vi "Wait-for-action-deposition.vi"(8 "error in (no error)":errorcluster, 11 "Object ref in":T2) -> (0 "error out":errorcluster, 2 "Action":T1=enum."Load deposition", 3 "Object ref out":T2)   [LabVIEW 2013, in "SLMControl.lvlib" / "SC-Main.lvclass"]
uses:
  SC-Main.lvclass
  Object-reference.ctl
  Deposition-actions.ctl
  SC-Main.lvclass/SC-Main.ctl
  Read Deposition queue.vi
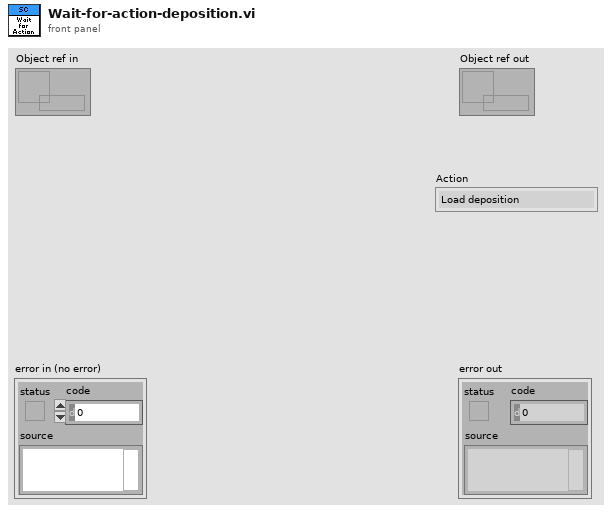
[diagram p1: front panel]
types:
  T1 = typedef "SLMControl.lvlib/SC-Main.lvclass/Deposition-actions.ctl" = enum16{"Idle", "Activate", "Load deposition", "Launch deposition", "Wait for deposition end", "Signal lasing", "Abort", "Reset", "Exit"}
  T2 = typedef "SLMControl.lvlib/SC-Main.lvclass/Object-reference.ctl" = refnum<data-value>
  T3 = typedef "BeamControl.lvlib/BC-Main.lvclass/Deposition-actions.ctl" = enum16{"Idle", "Activate", "Load deposition", "Launch deposition", "Wait for deposition end", "Signal lasing", "Abort", "Reset", "Exit"}
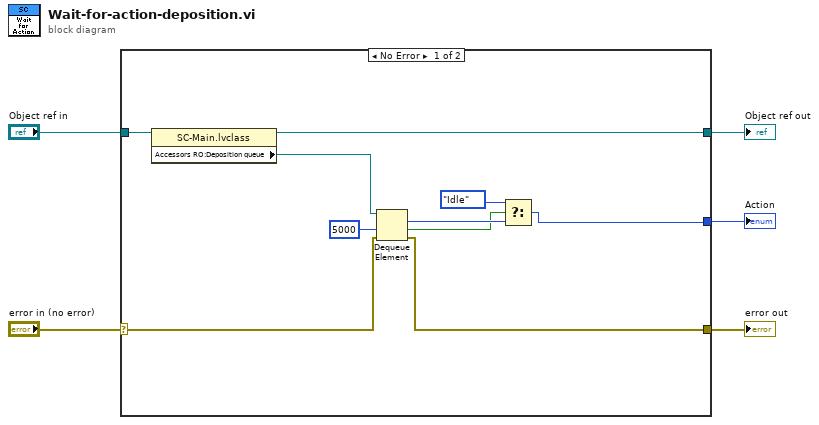
[diagram p0: block diagram]
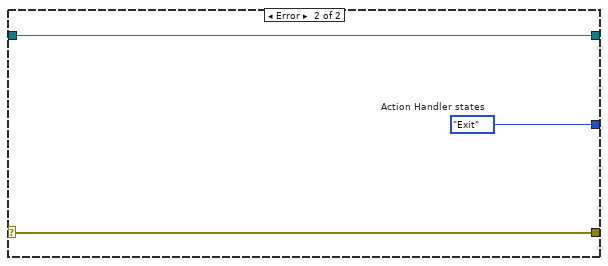
[diagram p2: hidden frame]
diagram:
  n1 = case shown="No Error" "error in (no error)" {
    selector: "error in (no error)" -> [w13 w18]
    tunnel: [w12 w18] -> w4
    tunnel: [w14 w17] -> w2
    tunnel: "Object ref in" -> [w15 w17]
    tunnel: [w6 w16] -> w1
    frame No Error {
      n2 = property class="SC-Main.lvclass"(reference=w15) -> (reference out=w14:T2, "Accessors RO:Deposition queue"=w11:refnum<queue>)  [unwired: 1 in, 1 out]
      n3 = Dequeue Element(queue=w11, timeout in ms (-1)=5000, error in (no error)=w13) -> (element=w9:T3, timed out?=w8:bool, error out=w12:errorcluster)  [unwired: 1 out]
      n4 = Select(t=Deposition-actions."Idle" ("Next execution"), s=w8, f=w9) -> (s? t:f=w6:T3)
    }
    frame Error {
      w16 = Deposition-actions."Exit"  # Action Handler states
    }
  }
  "error out" <- w4
  "Object ref out" <- w2
  "Action" <- w1
